vi "save_time_course.vi"(7 "stimulation type enum":T1, 8 "error in (no error)":errorcluster, 9 "base name":string, 10 "folder path":path, 11 "DataCollectionMG091001IntrinsicImaging in":refnum<class "DataCollectionMG091001IntrinsicImaging.lvclass">) -> (0 "error out":errorcluster, 3 "DataCollectionMG091001IntrinsicImaging out":refnum<class "DataCollectionMG091001IntrinsicImaging.lvclass">)   [LabVIEW 2010, in "DataCollectionMG091001IntrinsicImaging.lvclass"]
uses:
  DataCollectionMG091001IntrinsicImaging.lvclass
  sweep_part_enum.ctl
  common/classes/ImageCollection/ImageCollection/ImageCollection.lvclass
  DataCollectionMG091001IntrinsicImaging.lvclass/DataCollectionMG091001IntrinsicImaging.ctl
  common/classes/ImageCollection/ImageCollection/add_mode_enum.ctl
  common/classes/ErrorController/ErrorController/class_data.vi
  common/classes/ErrorController/ErrorController/ErrorController.lvclass
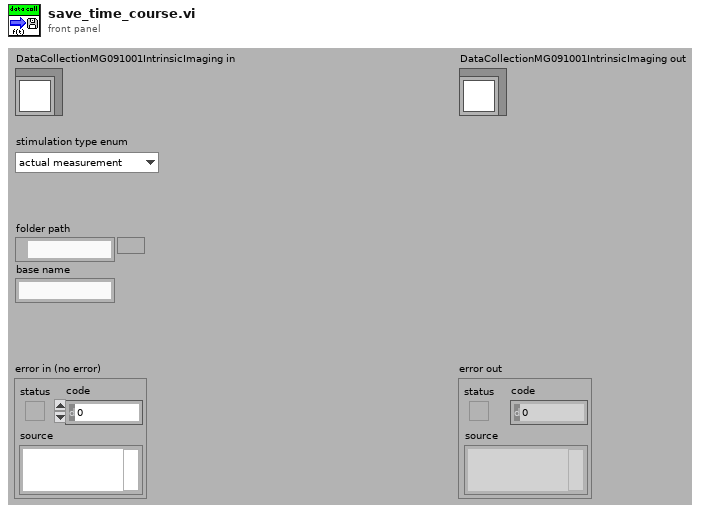
[diagram p1: front panel]
types:
  T1 = typedef "DataCollectionMG091001IntrinsicImaging.lvclass/sweep_part_enum.ctl" = enum16{"actual measurement", "control"}
  T2 = typedef "ImageCollection.lvclass/add_mode_enum.ctl" = enum16{"instance", "copy"}
  T3 = typedef "DataCollectionMG091001IntrinsicImaging.lvclass/individual_sweeps_saving_enum.ctl" = enum32{"autosave sweeps on the fly", "save individual sweeps", "don't save individual sweeps"}
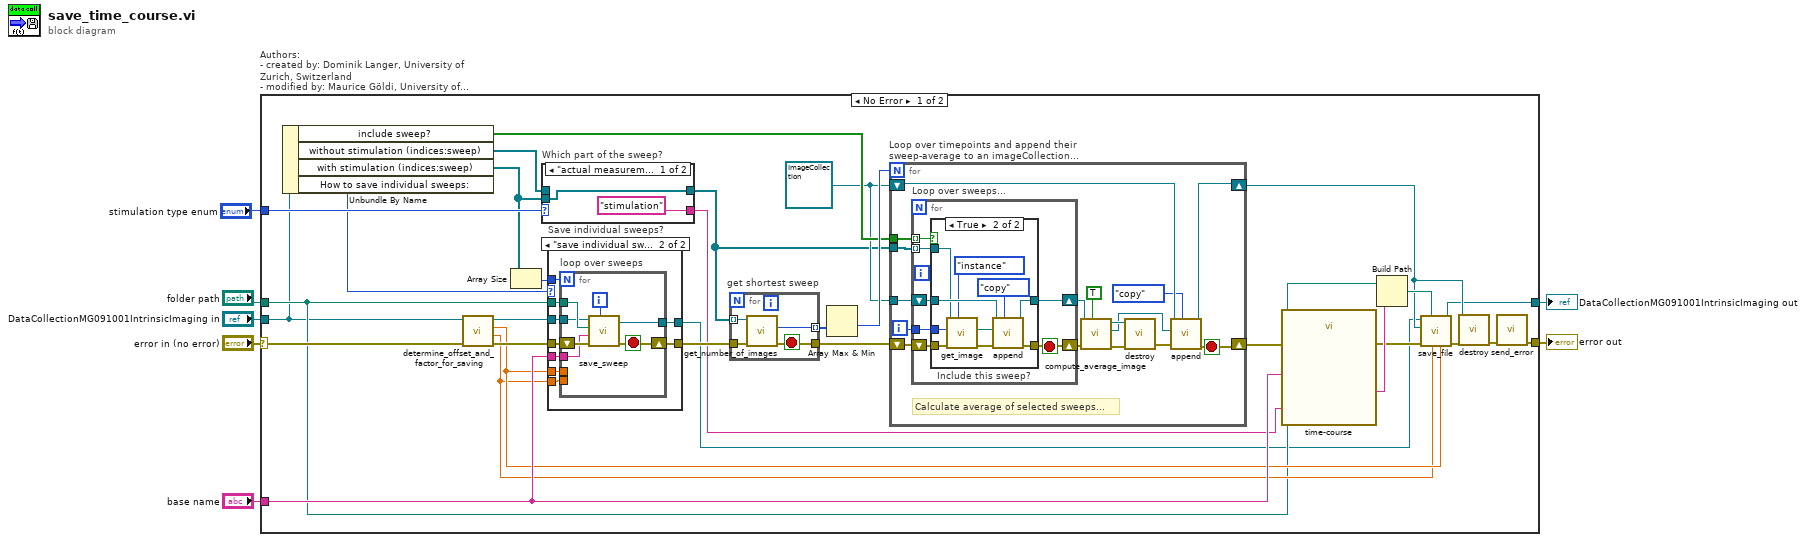
[diagram p0: block diagram]
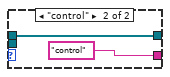
[diagram p2: hidden frame]
diagram:
  n1 = case "Authors: \n- created by: Dominik Langer, University of Zurich, Switzerland\n- modified by: Maurice Göldi, University of Zurich, Switzerland" shown="No Error" "error in (no error)" {
    selector: "error in (no error)" -> [w18 w101]
    tunnel: [w20 w101] -> w6
    tunnel: [w24 w100] -> w4
    tunnel: "DataCollectionMG091001IntrinsicImaging in" -> [w12 w100]
    tunnel: "stimulation type enum" -> [w27 _]
    tunnel: "folder path" -> [w14 _]
    tunnel: "base name" -> [w23 _]
    frame No Error {
      w25 = refnum<class "ImageCollection.lvclass"> refnum ("ImageCollection.lvclass")
      n2 = Unbundle By Name(w12) -> ("include sweep?"=w28:bool[], "without stimulation (indices:sweep)"=w26:refnum<class "ImageCollection.lvclass">[], "with stimulation (indices:sweep)"=w8:refnum<class "ImageCollection.lvclass">[], "How to save individual sweeps:"=w11:T3)
      n3 = call-dynamic "determine_offset_and_factor_for_saving.vi"("error in (no error)"=w18, "DataCollectionMG091001IntrinsicImaging in"=w12) -> ("error out"=w17:errorcluster, "factor"=w15:dbl, "offset"=w16:dbl, "DataCollectionMG091001IntrinsicImaging out"=w19:refnum<class "DataCollectionMG091001IntrinsicImaging.lvclass">)  [unwired: 6 in]
      n4 = Array Size(array=w8) -> (size(s)=w9:i32)
      n5 = case "Which part of the sweep?" shown="\"actual measurement\", Default" w27 {
        tunnel: w26 -> [_ w42]
        tunnel: w8 -> [w40 _]
        tunnel: [w40 w42] -> w13
        tunnel: ["stimulation" "control"] -> w22
        frame "actual measurement", Default {
        }
        frame "control" {
        }
      }
      n6 = case "Save individual sweeps?" shown="\"save individual sweeps\"" w11 {
        tunnel: w17 -> [w43 w53]
        tunnel: [w43 w52] -> w31
        tunnel: w14 -> [_ w51]
        tunnel: w23 -> [_ w50]
        tunnel: w19 -> [w44 w49]
        tunnel: [w44 w48] -> w10
        tunnel: w16 -> [_ w47]
        tunnel: w15 -> [_ w46]
        tunnel: w9 -> [_ w45]
        frame Default {
        }
        frame "save individual sweeps" {
          n7 = for "loop over sweeps" {
            N: w45 -> [_]
            tunnel: w51 -> [w60]
            tunnel: w50 -> [w54]
            tunnel: w49 -> [w57]
            tunnel: [w55] -> w48
            tunnel: w47 -> [_]
            tunnel: w46 -> [_]
            shift-right: [w58] -> w52
            shift-left: w53 -> [w59]
            i -> [w56]
            stop <- w58 stop-if-true
            n8 = call-dynamic "save_sweep.vi"("sweep index"=w56, "error in (no error)"=w59, "base name"=w54, "folder path"=w60, "DataCollectionMG091001IntrinsicImaging in"=w57) -> ("error out"=w58:errorcluster, "DataCollectionMG091001IntrinsicImaging out"=w55:refnum<class "DataCollectionMG091001IntrinsicImaging.lvclass">)  [unwired: 5 in]
          }
        }
      }
      n9 = for "get shortest sweep" {
        tunnel: w13 -> [w63] mode=indexing
        tunnel: [w62] -> w30 mode=indexing
        tunnel: w31 -> [w64]
        tunnel: [w61] -> w38
        stop <- w61 stop-if-true
        n10 = call-dynamic "get_number_of_images.vi"("error in (no error)"=w64, "ImageCollection in"=w63) -> ("error out"=w61:errorcluster, "size"=w62:i32)  [unwired: 7 in, 1 out]
      }
      n11 = Array Max & Min(array=w30) -> (min value=w29:i32)  [unwired: 3 out]
      n12 = for "Loop over timepoints and append their sweep-average to an imageCollection..." {
        N: w29 -> [_]
        tunnel: w28 -> [w75]
        tunnel: w13 -> [w74]
        shift-right: [w69] -> w32
        shift-left: w25 -> [w71]
        tunnel: w25 -> [w67]
        shift-right: [w65] -> w37
        shift-left: w38 -> [w68]
        i -> [w66]
        stop <- w65 stop-if-true
        # "Calculate average of selected sweeps..."
        n13 = for "Loop over sweeps..." {
          shift-right: [w87] -> w78
          shift-left: w67 -> [w86]
          tunnel: w75 -> [w83] mode=indexing
          tunnel: w74 -> [w84] mode=indexing
          tunnel: w66 -> [w82]
          shift-right: [w81] -> w80
          shift-left: w68 -> [w85]
          stop <- w81 stop-if-true
          n14 = case "Include this sweep?" shown="True" w83 {
            tunnel: [w88 w99] -> w81
            tunnel: [w89 w98] -> w87
            tunnel: w86 -> [w89 w96]
            tunnel: w85 -> [w88 w94]
            tunnel: w84 -> [_ w92]
            tunnel: w82 -> [_ w90]
            frame False {
            }
            frame True {
              n15 = call-dynamic "get_image.vi"("get image as..."=add_mode_enum."instance", "error in (no error)"=w94, "index"=w90, "ImageCollection in"=w92) -> ("error out"=w95:errorcluster, "Image.lvclass"=w93:refnum<class "Image.lvclass">)  [unwired: 5 in, 1 out]
              n16 = call-dynamic "append.vi"("add mode"=add_mode_enum."copy", "error in (no error)"=w95, "Image.lvclass"=w93, "ImageCollection in"=w96) -> ("error out"=w99:errorcluster, "ImageCollection out"=w98:refnum<class "ImageCollection.lvclass">)  [unwired: 5 in, 1 out]
            }
          }
        }
        n17 = call-dynamic "compute_average_image.vi"("all?"=TRUE, "error in (no error)"=w80, "ImageCollection in"=w78) -> ("error out"=w79:errorcluster, "averaged image"=w72:refnum<class "Image.lvclass">, "ImageCollection out"=w77:refnum<class "ImageCollection.lvclass">)  [unwired: 6 in]
        n18 = call-dynamic "destroy.vi"("error in (no error)"=w79, "ImageCollection in"=w77) -> ("error out"=w73:errorcluster)  [unwired: 8 in, 1 out]
        n19 = call-dynamic "append.vi"("add mode"=add_mode_enum."copy", "error in (no error)"=w73, "Image.lvclass"=w72, "ImageCollection in"=w71) -> ("error out"=w65:errorcluster, "ImageCollection out"=w69:refnum<class "ImageCollection.lvclass">)  [unwired: 5 in, 1 out]
      }
      n20 = call "time-course"("base"=w23, "type"=w22, "error in (no error)"=w37) -> ("Result"=w36:string, "error out"=w35:errorcluster)  [unwired: 11 in]
      n21 = Build Path(base path=w14, name or relative path=w36) -> (appended path=w34:path)
      n22 = call-dynamic "save_file.vi"("offset"=w16, "multiplication factor"=w15, "path"=w34, "error in (no error)"=w35, "ImageCollection in"=w32, "DataCollectionDL090215 in"=w10) -> ("error out"=w33:errorcluster, "DataCollectionDL090215 out"=w24:refnum<class "DataCollectionMG091001IntrinsicImaging.lvclass">)  [unwired: 4 in]
      n23 = call-dynamic "destroy.vi"("error in (no error)"=w33, "ImageCollection in"=w32) -> ("error out"=w21:errorcluster)  [unwired: 8 in, 1 out]
      n24 = call "send_error.vi"("error in (no error)"=w21) -> ("error out"=w20:errorcluster)  [unwired: 10 in]
    }
    frame Error {
    }
  }
  "error out" <- w6
  "DataCollectionMG091001IntrinsicImaging out" <- w4
